vi "Write Multiple Holding Registers.vi"(8 "error in (no error)":errorcluster, 9 "registers to write":u16[](array[numeric]), 10 "starting address":u16, 11 "Modbus instance in":refnum<class "Modbus API.lvclass">) -> (0 "error out":errorcluster, 3 "Modbus instance out":refnum<class "Modbus API.lvclass">)   [LabVIEW 2020, in "SubVIs.lvlib" / "Modbus API.lvclass"]
doc: "Writes <B>registers to write</B> starting at <B>starting address</B> to the device holding registers."
uses:
  <vilib>/Modbus/subvis/Modbus API/Modbus API.lvclass
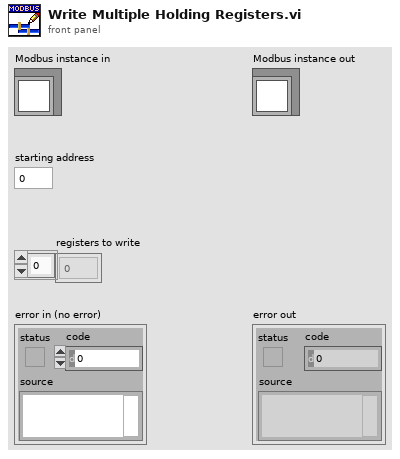
[diagram p1: front panel]
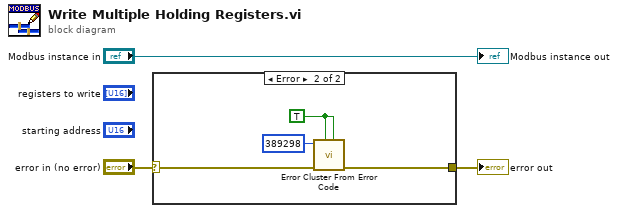
[diagram p0: block diagram]
diagram:
  n1 = case shown="Error" "error in (no error)" {
    selector: "error in (no error)" -> [w4 w8]
    tunnel: [w4 w7] -> w1
    frame No Error {
    }
    frame Error {
      w5 = TRUE ("show call chain? (False)")
      n2 = call <vilib>:"Error Cluster From Error Code.vi"("is warning? (False)"=w5, "show call chain? (False)"=w5, "error in (no error)"=w8, "error code (0)"=389298) -> ("error out"=w7:errorcluster)  [unwired: 5 in]
    }
  }
  "error out" <- w1
  "Modbus instance out" <- "Modbus instance in"
